vi "ReferenceSet.vi"(6 "设置参数":string, 7 "参数查询(0)/设置(1)":bool, 8 "error in (no error)":errorcluster caption="错误输入（无错误）", 9 "REFERENCE命令子系统":string(combo), 10 "参考通道":string(combo), 11 "VISA资源名称":refnum<visa-resource-name>) -> (0 "error out":errorcluster caption="错误输出", 1 "查询返回字节数":u32, 2 "查询返回":string, 3 "VISA资源名称 2":refnum<visa-resource-name>)   [LabVIEW 2018]
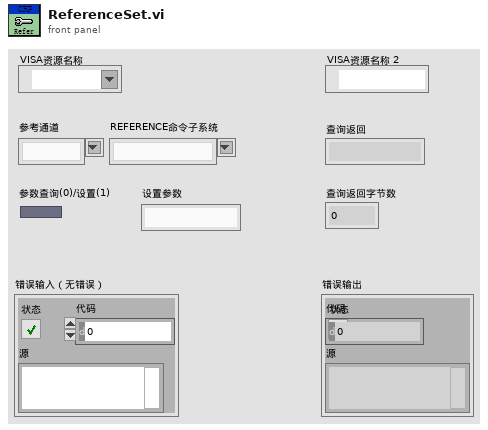
[diagram p1: front panel]
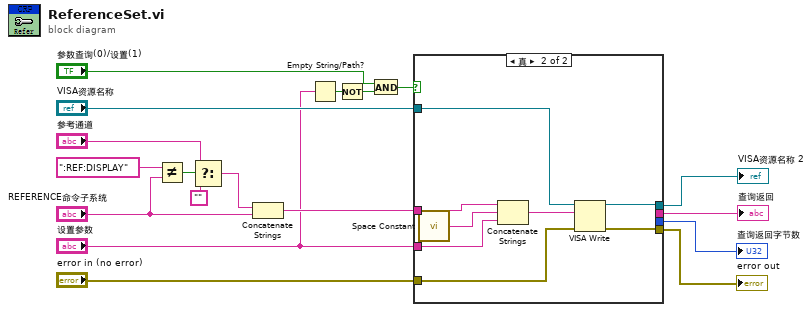
[diagram p0: block diagram]
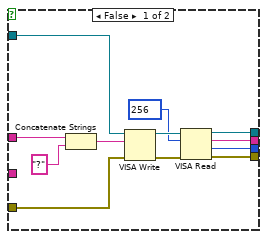
[diagram p2: hidden frame]
diagram:
  n1 = Not Equal?(x=":REF:DISPLAY", y="REFERENCE命令子系统") -> (x != y?=w7:bool)
  n2 = Select(t="参考通道", s=w7, f="") -> (s? t:f=w6:string)
  n3 = Concatenate Strings(w6, "REFERENCE命令子系统") -> (w2:string)
  n4 = Empty String/Path?(string/path="设置参数") -> (empty?=w13:bool)
  n5 = Not(x=w13) -> (.not. x?=w10:bool)
  n6 = And(x="参数查询(0)/设置(1)", y=w10) -> (x .and. y?=w15:bool)
  n7 = case shown="真" w15 {
    tunnel: "设置参数" -> [_ w37]
    tunnel: "error in (no error)" -> [w20 w32]
    tunnel: [w26 w34] -> w17
    tunnel: [w25 _] -> w12
    tunnel: [w24 w35] -> w16
    tunnel: w2 -> [w23 w36]
    tunnel: "VISA资源名称" -> [w21 w31]
    tunnel: [w19 _] -> w11
    frame False {
      n8 = Concatenate Strings(w23, "?") -> (w30:string)
      n9 = VISA Write(VISA resource name=w21, write buffer=w30, error in (no error)=w20) -> (VISA resource name out=w28:refnum<visa-resource-name>, error out=w29:errorcluster)  [unwired: 1 out]
      n10 = VISA Read(VISA resource name=w28, byte count=u32 256 ("字节总数"), error in (no error)=w29) -> (VISA resource name out=w24:refnum<visa-resource-name>, read buffer=w25:string, return count=w19:u32, error out=w26:errorcluster)
    }
    frame True {
      n11 = call <vilib>:"Space Constant.vi"() -> ("String"=w38:string)
      n12 = Concatenate Strings(w36, w38, w37) -> (w33:string)
      n13 = VISA Write(VISA resource name=w31, write buffer=w33, error in (no error)=w32) -> (VISA resource name out=w35:refnum<visa-resource-name>, error out=w34:errorcluster)  [unwired: 1 out]
    }
  }
  "error out" <- w17
  "VISA资源名称 2" <- w16
  "查询返回" <- w12
  "查询返回字节数" <- w11
